vi "test20-RegisterStatusAsInterruptFromNonCSM.vi"(8 "error in (no error)":errorcluster, 11 "TestCase in":refnum<class "testcase-CSMBroadcast.lvclass">) -> (0 "error out":errorcluster, 3 "TestCase out":refnum<class "testcase-CSMBroadcast.lvclass">)   [LabVIEW 2017, in "testcase-CSMBroadcast.lvclass"]
uses:
  testcase-CSMBroadcast.lvclass
  src/user.lib/_NEVSTOP/Communicable State Machine(CSM)/AdvanceAPI/CSM - Broadcast Message Type.ctl
  <vilib>/addons/_JKI Toolkits/VI Tester/TestCase.llb/TestCase.lvclass
  src/user.lib/_NEVSTOP/Communicable State Machine(CSM)/Communicable State Machine.lvlib
  CSM/CSM-Testcase.lvlib
  C:/Program Files (x86)/National Instruments/LabVIEW 2017/vi.lib/addons/_JKI Toolkits/VI Tester/TestCase.llb/TestCase.lvclass
panel:
  out "output cluster":T1
  out "LoopCount":i32
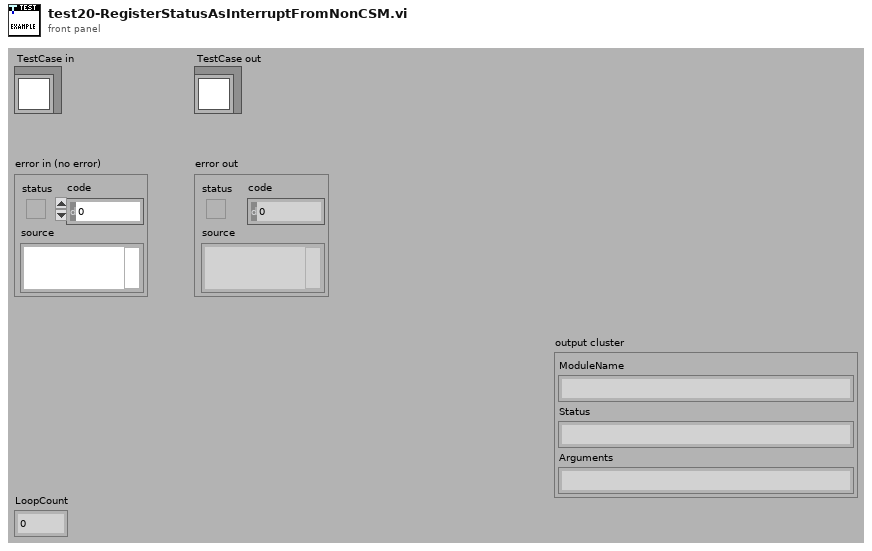
[diagram p1: front panel]
types:
  T1 = cluster{"ModuleName":string, "Status":string, "Arguments":string}
  T2 = typedef "Communicable State Machine.lvlib/CSM - Broadcast Message Type.ctl" = enum16{"<Null>", "Status", "Interrupt"}
  T3 = cluster{"Status Event":refnum<user-event>, "Interrupt Event":refnum<user-event>}
  T4 = cluster{"cluster":cluster{"ModuleName":string, "Status":string, "Arguments":string}}
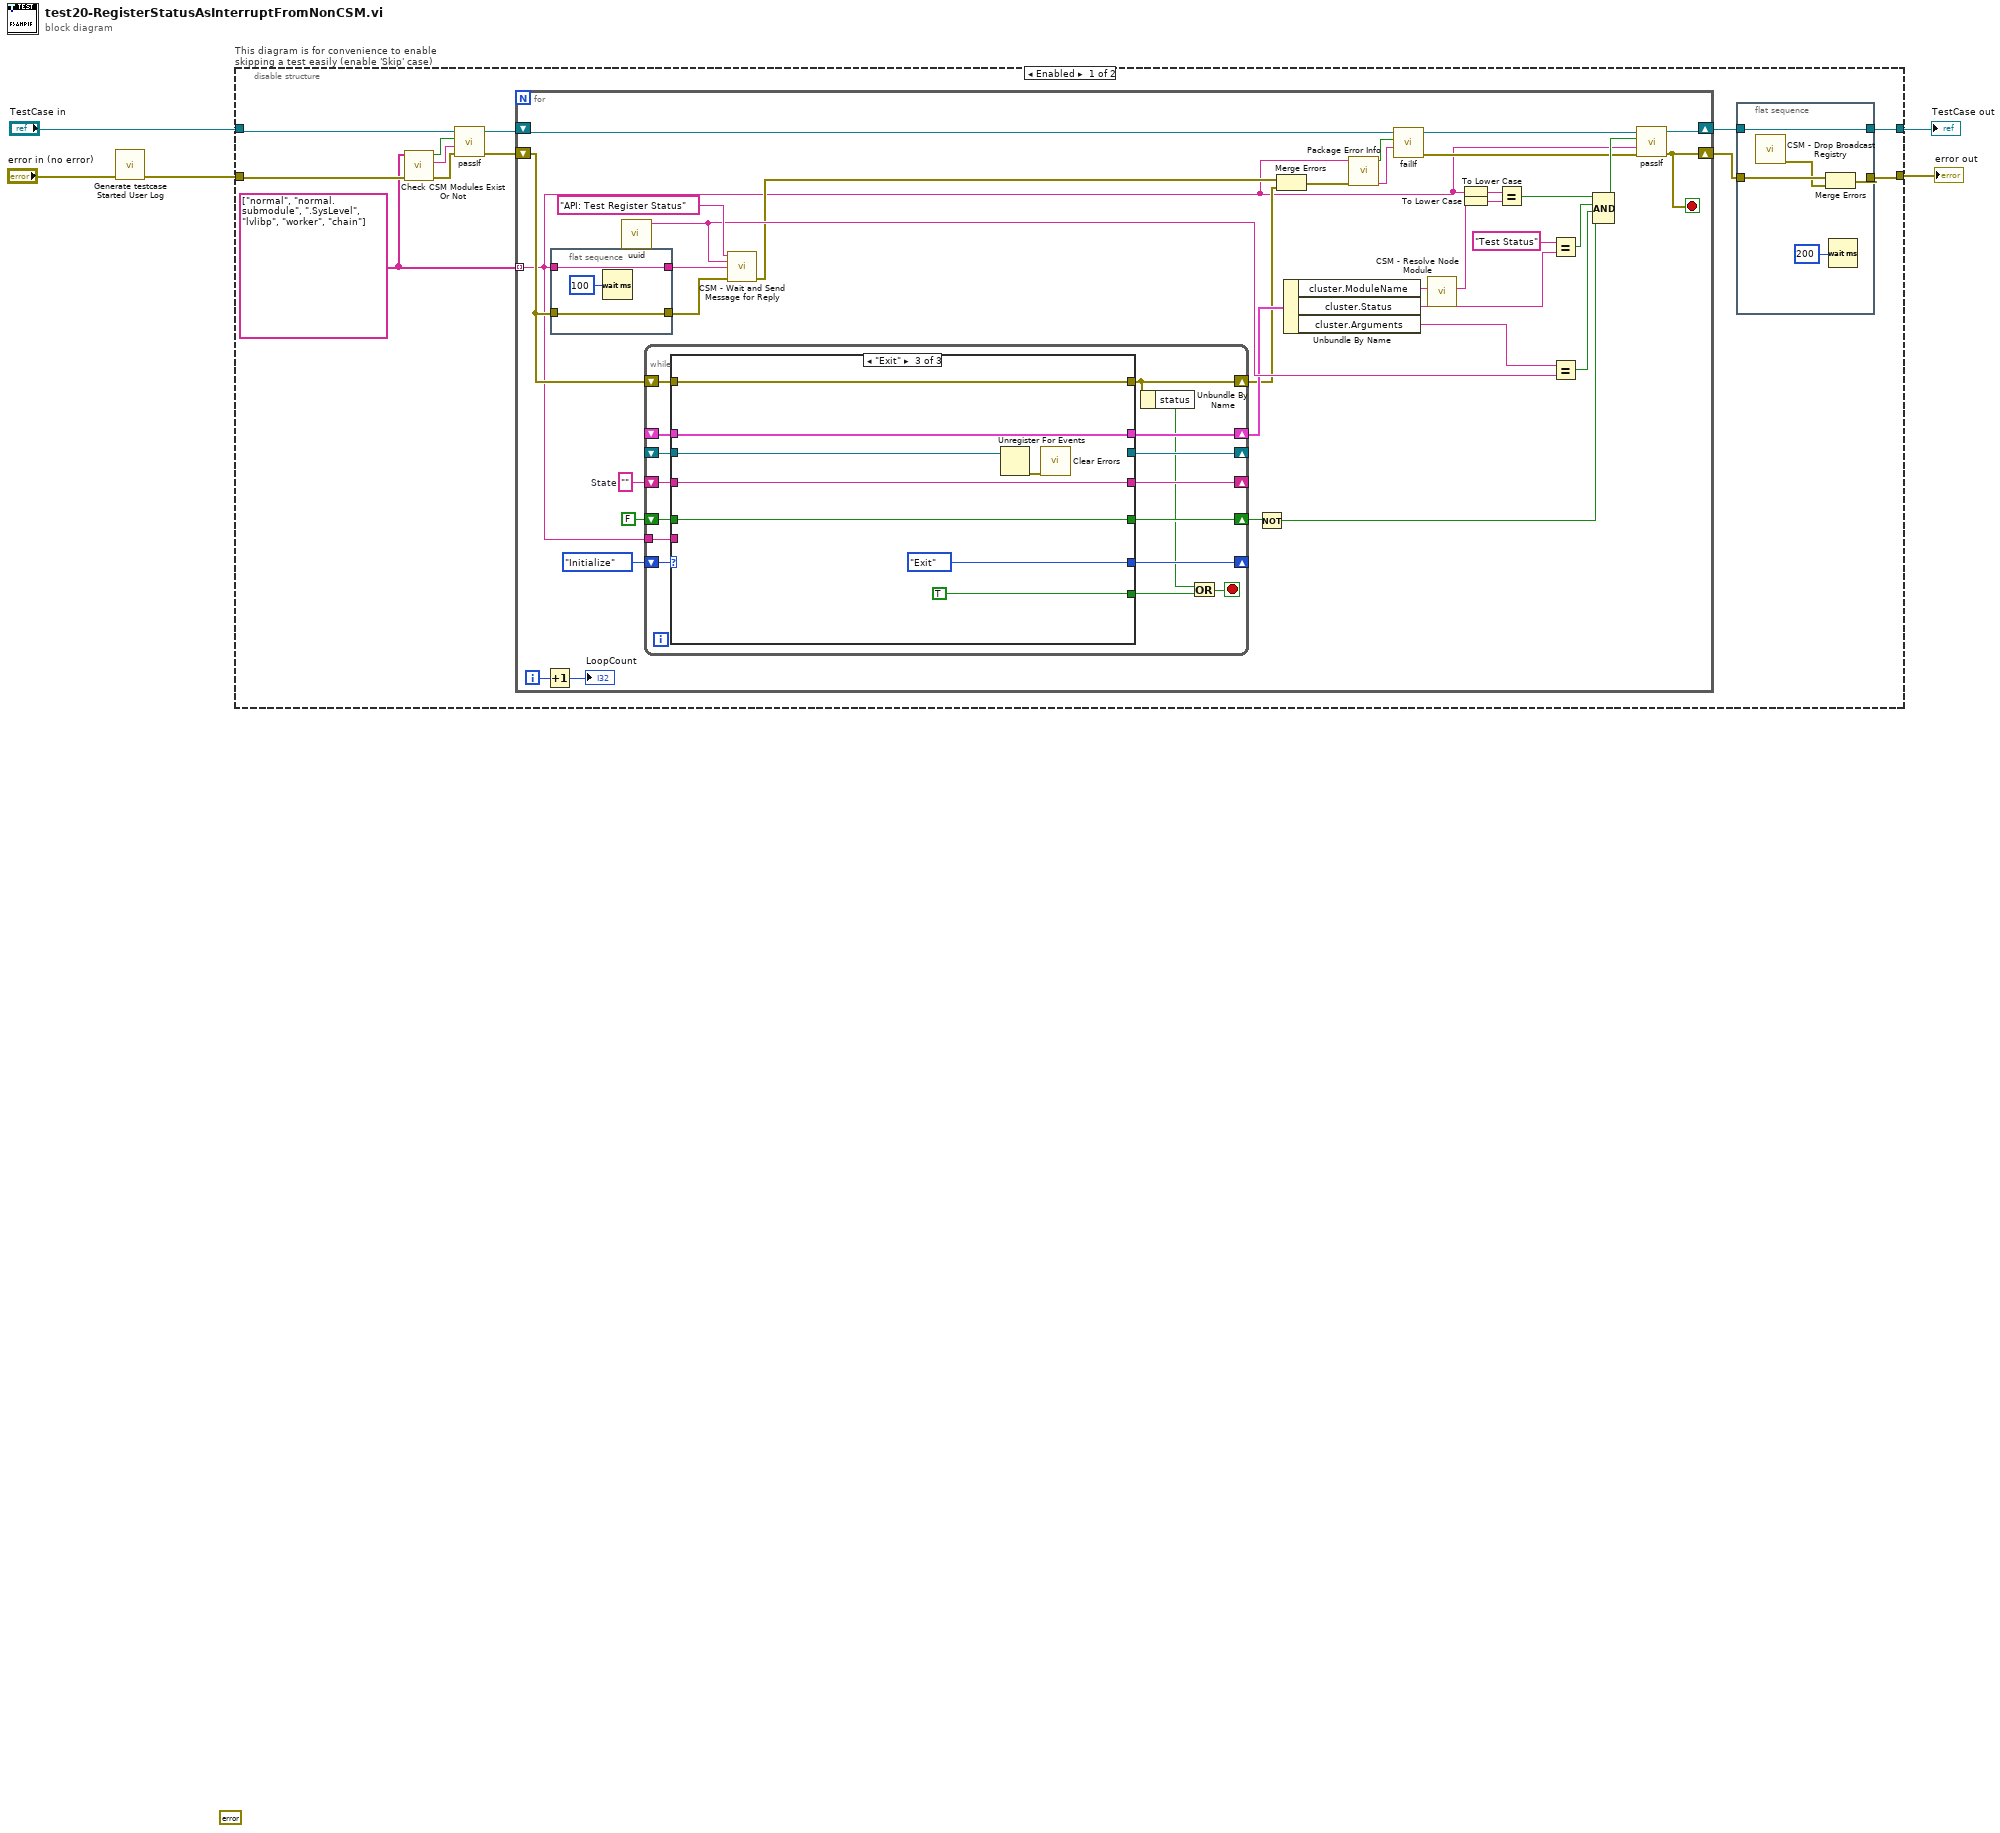
[diagram p0: block diagram]
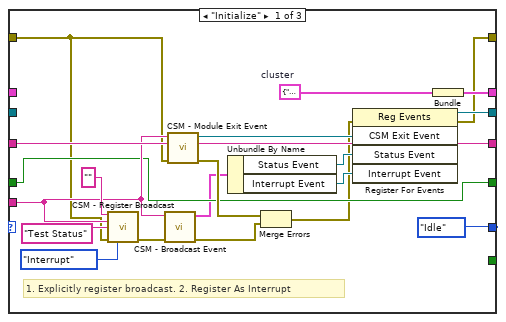
[diagram p2: hidden frame]
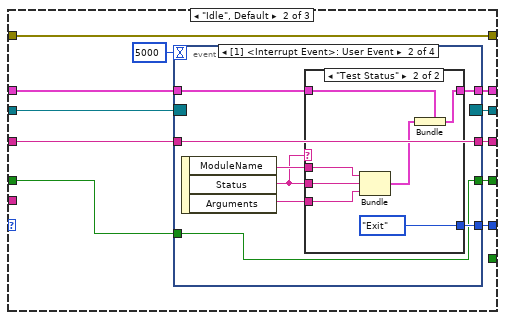
[diagram p3: hidden frame]
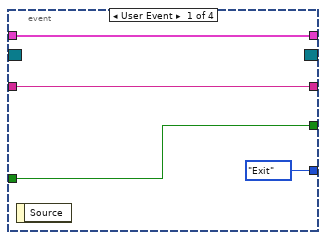
[diagram p4: hidden frame]
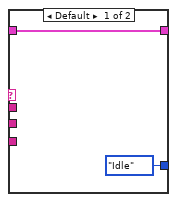
[diagram p5: hidden frame]
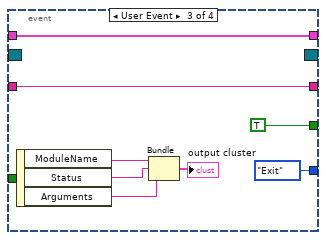
[diagram p6: hidden frame]
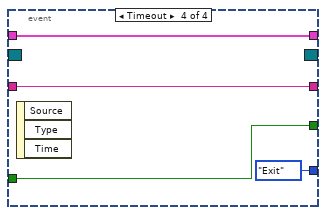
[diagram p7: hidden frame]
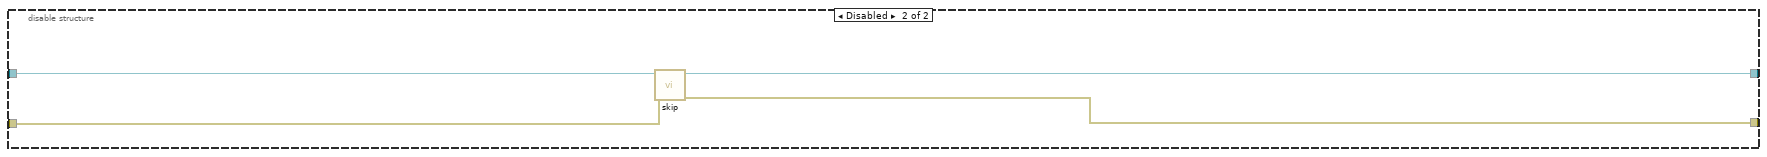
[diagram p8: hidden frame]
diagram:
  (unwired) errorcluster {"status"=FALSE, "code"=0, "source"=""} ("error out")
  n1 = call "Generate testcase Started User Log.vi"("Error In"="error in (no error)") -> ("error out"=w1:errorcluster)  [unwired: 10 in]
  n2 = disable-structure "This diagram is for convenience to enable skipping a test easily (enable 'Skip' case)" shown="Enabled" {
    disable-tunnel: "TestCase in" -> [w14 w152]
    disable-tunnel: [w8 w150] -> w3
    disable-tunnel: [w6 w151] -> w2
    disable-tunnel: w1 -> [w12 w149]
    frame Enabled {
      w10 = string[] ["normal", "normal.submodule", ".SysLevel", "lvlibp", "worker", "chain"]
      n3 = call "Check CSM Modules Exist Or Not.vi"("error in"=w12, "CSM names in"=w10) -> ("error out"=w15:errorcluster, "Debug string"=w16:string, "All Modules Exist?"=w17:bool)  [unwired: 7 in]
      n4 = call-dynamic "passIf.vi"("error in (no error)"=w15, "message (\"\")"=w16, "pass"=w17, "TestCase in"=w14) -> ("error out"=w11:errorcluster, "TestCase out"=w13:refnum<class "testcase-CSMBroadcast.lvclass">)  [unwired: 6 in]
      n5 = for {
        shift-right: [w49] -> w9
        shift-left: w13 -> [w29]
        tunnel: w10 -> [w23] mode=indexing
        shift-right: [w42] -> w7
        shift-left: w11 -> [w32]
        i -> [w44]
        stop <- w42 stop-if-true
        w56 = ""  # State
        n6 = Increment(x=w44) -> (x+1=→"LoopCount":i32)
        n7 = flat-sequence {
          tunnel: w23 -> [w60]
          tunnel: [w60] -> w54
          tunnel: [w58] -> w33
          tunnel: w32 -> [w58]
          frame #0 {
            n8 = Wait (ms)(milliseconds to wait=u32 100) -> ()  [unwired: 1 out]
          }
        }
        n9 = call "uuid.vi"() -> ("UUID"=w51:string)  [unwired: 11 in]
        n10 = while {
          shift-right: [w75] -> _
          shift-left: enum16{"Idle", "Initialize", "Exit"}."Initialize" -> [w76]
          shift-right: [w73] -> _
          shift-left: w56 -> [w74]
          shift-right: [w72] -> _
          shift-left: _ -> [w71]
          shift-right: [w70] -> w41
          shift-left: _ -> [w69]
          tunnel: w23 -> [w68]
          shift-right: [w67] -> w36
          shift-left: FALSE -> [w66]
          shift-right: [w62] -> w25
          shift-left: w32 -> [w65]
          stop <- w64 stop-if-true
          n11 = case shown="\"Exit\"" w76 {
            tunnel: [enum16{"Idle", "Initialize", "Exit"}."Idle" w107 enum16{"Idle", "Initialize", "Exit"}."Exit"] -> w75
            tunnel: [_ _ TRUE] -> w63
            tunnel: w74 -> [w95 w105 w146]
            tunnel: [w95 w106 w146] -> w73
            tunnel: [w93 w103 _] -> w72
            tunnel: w71 -> [_ w104 w145]
            tunnel: [w92 w101 w143] -> w70
            tunnel: w69 -> [_ w102 w143]
            tunnel: w68 -> [w85 _ _]
            tunnel: [w82 w99 w142] -> w67
            tunnel: w66 -> [w82 w98 w142]
            tunnel: w65 -> [w79 w97 w141]
            tunnel: [w77 w97 w141] -> w62
            frame "Initialize" {
              w91 = T1 {"ModuleName"="", "Status"="", "Arguments"=""}  # cluster
              # "1. Explicitly register broadcast. 2. Register As Interrupt"
              n12 = call "CSM - Register Broadcast.vi"("CSM Name(Empty for Broadcast Event)"="", "Source CSM Name (* as Default)"=w85, "Trigger"="Test Status" ("State"), "Error In"=w79, "Priority (No Change)"=CSM_-_Broadcast_Message_Type."Interrupt" ("Priority(No Change)")) -> ("error out"=w87:errorcluster)  [unwired: 9 in, 1 out]
              n13 = call "CSM - Broadcast Event.vi"("Error In"=w87, "CSM Module"=w85) -> ("error out"=w89:errorcluster, "Broadcast Event"=w81:T3)  [unwired: 7 in, 1 out]
              n14 = call "CSM - Module Exit Event.vi"("Error In"=w79, "Name (\"\" to Use UUID) In"=w85) -> ("error out"=w90:errorcluster, "CSM Exit Event"=w94:refnum<user-event>)  [unwired: 7 in, 1 out]
              n15 = Unbundle By Name(w81) -> ("Status Event"=w84:refnum<user-event>, "Interrupt Event"=w83:refnum<user-event>)
              n16 = Merge Errors(w90, w89) -> (w78:errorcluster)
              n17 = register-events(error in=w78, w94, w84, w83) -> (reference out=w93:refnum<event-registration>, error out=w77:errorcluster)  [unwired: 1 in]
              n18 = Bundle("cluster"=w91) -> (w92:T4)  [unwired: 1 in]
            }
            frame "Idle", Default {
              n19 = event shown="[1] <Interrupt Event>: User Event" {
                selector: w104 -> [_ _ _ _]
                dyn-events: [_ _ _ _] -> w103
                timeout: 5000 -> [_ _ _ _]
                tunnel: [enum16{"Idle", "Initialize", "Exit"}."Exit" w118 enum16{"Idle", "Initialize", "Exit"}."Exit" enum16{"Idle", "Initialize", "Exit"}."Exit"] -> w107
                tunnel: w105 -> [w111 w119 w136 w140]
                tunnel: [w111 w119 w136 w140] -> w106
                tunnel: w102 -> [w109 w115 w135 w139]
                tunnel: [w109 w114 w135 w139] -> w101
                tunnel: [w108 w112 TRUE w137] -> w99
                tunnel: w98 -> [w108 w112 _ w137]
                event User Event {
                  n20 = event-data() -> ()  [unwired: 1 in, 1 out]
                }
                event User Event {
                  n21 = event-data() -> ("ModuleName"=w117:string, "Status"=w113:string, "Arguments"=w116:string)  [unwired: 1 in]
                  n22 = case shown="\"Test Status\"" w113 {
                    tunnel: [enum16{"Idle", "Initialize", "Exit"}."Idle" enum16{"Idle", "Initialize", "Exit"}."Exit"] -> w118
                    tunnel: w117 -> [_ w127]
                    tunnel: w113 -> [_ w126]
                    tunnel: w116 -> [_ w125]
                    tunnel: w115 -> [w121 w124]
                    tunnel: [w121 w122] -> w114
                    frame Default {
                    }
                    frame "Test Status" {
                      n23 = Bundle("ModuleName"=w127, "Status"=w126, "Arguments"=w125) -> (w123:T1)  [unwired: 1 in]
                      n24 = Bundle(cluster=w124, "cluster"=w123) -> (w122:T4)
                    }
                  }
                }
                event User Event {
                  n25 = event-data() -> ("ModuleName"=w132:string, "Status"=w131:string, "Arguments"=w130:string)  [unwired: 1 in]
                  n26 = Bundle("ModuleName"=w132, "Status"=w131, "Arguments"=w130) -> (→"output cluster":T1)  [unwired: 1 in]
                }
                event Timeout {
                  n27 = event-data() -> ()  [unwired: 1 in, 3 out]
                }
              }
            }
            frame "Exit" {
              n28 = Unregister For Events(event registration refnum=w145) -> (error out=w144:errorcluster)  [unwired: 1 in]
              n29 = call <vilib>:"Clear Errors.vi"("error in (no error)"=w144) -> ()  [unwired: 5 in, 2 out]
            }
          }
          n30 = Unbundle By Name(w62) -> ("status"=w61:bool)
          n31 = Or(x=w61, y=w63) -> (x .or. y?=w64:bool)
        }
        n32 = call "CSM - Wait and Send Message for Reply.vi"("State"="API: Test Register Status", "Arguments (\"\")"=w51, "Target Module"=w54, "Error In (No Error)"=w33) -> ("error out"=w26:errorcluster)  [unwired: 8 in, 3 out]
        n33 = Not(x=w36) -> (.not. x?=w35:bool)
        n34 = Merge Errors(w26, w25) -> (w24:errorcluster)
        n35 = Unbundle By Name(w41) -> ("cluster.ModuleName"=w39:string, "cluster.Status"=w52:string, "cluster.Arguments"=w50:string)
        n36 = call "Package Error Info.vi"("error in"=w24, "String in"=w23) -> ("packed error info out"=w30:string, "error status"=w31:bool)  [unwired: 8 in]
        n37 = call-dynamic "failIf.vi"("message (\"\")"=w30, "fail"=w31, "TestCase in"=w29) -> ("error out"=w27:errorcluster, "TestCase out"=w28:refnum<class "testcase-CSMBroadcast.lvclass">)  [unwired: 7 in]
        n38 = call "CSM - Resolve Node Module.vi"("Node Name"=w39) -> ("CSM Module Name"=w37:string)  [unwired: 10 in]
        n39 = To Lower Case(string=w23) -> (all lower case string=w40:string)
        n40 = To Lower Case(string=w37) -> (all lower case string=w38:string)
        n41 = Equal?(x=w40, y=w38) -> (x = y?=w48:bool)
        n42 = Equal?(x="Test Status" ("State"), y=w52) -> (x = y?=w47:bool)
        n43 = Equal?(x=w50, y=w51) -> (x = y?=w46:bool)
        n44 = Compound Arithmetic op=AND(w48, w47, w46, w35) -> (w45:bool)
        n45 = call-dynamic "passIf.vi"("error in (no error)"=w27, "message (\"\")"=w23, "pass"=w45, "TestCase in"=w28) -> ("error out"=w42:errorcluster, "TestCase out"=w49:refnum<class "testcase-CSMBroadcast.lvclass">)  [unwired: 6 in]
      }
      n46 = flat-sequence {
        tunnel: w7 -> [w22]
        tunnel: [w21] -> w6
        tunnel: w9 -> [w19]
        tunnel: [w19] -> w8
        frame #0 {
          n47 = call "CSM - Drop Broadcast Registry.vi"() -> ("error out"=w20:errorcluster)  [unwired: 15 in]
          n48 = Merge Errors(w22, w20) -> (w21:errorcluster)
          n49 = Wait (ms)(milliseconds to wait=u32 200) -> ()  [unwired: 1 out]
        }
      }
    }
    frame Disabled {
      # "skip test result while test is under development"
      n50 = call <vilib>:"skip.vi"("error in (no error)"=w149, "TestCase in"=w152) -> ("error out"=w151:errorcluster, "TestCase out"=w150:refnum<class "testcase-CSMBroadcast.lvclass">)  [unwired: 8 in]
    }
  }
  "error out" <- w2
  "TestCase out" <- w3
